vi "IMU garbo.vi"(5 "Align?":bool, 6 "Velocity Data":dbl[](array[numeric]), 7 "PID gains":T1={"proportional gain (Kc)"=1.0, "integral time (Ti, min)"=0.01, "derivative time (Td, min)"=0.0} {"derivative time (Td, min)" format="%.3f"; "integral time (Ti, min)" format="%.3f"; "proportional gain (Kc)" format="%.3f"}, 8 "Numeric":dbl, 9 "Angular Data (Relative)":dbl[](array[numeric]), 10 "Angle to Get":dbl, 11 "Iterations":dbl) -> (0 "Current Velocity":dbl, 1 "output":dbl, 2 "output 2":dbl, 3 "IPCed":dbl)   [LabVIEW 2019]
uses:
  <vilib>/addons/control/pid/pid.llb/PID (DBL).vi
  <vilib>/addons/control/pid/NI_PID_pid.lvlib
panel:
  out "Error":dbl
  out "Waveform Chart":cluster{"Current Angle 2":dbl, "Numeric":dbl}(graph)
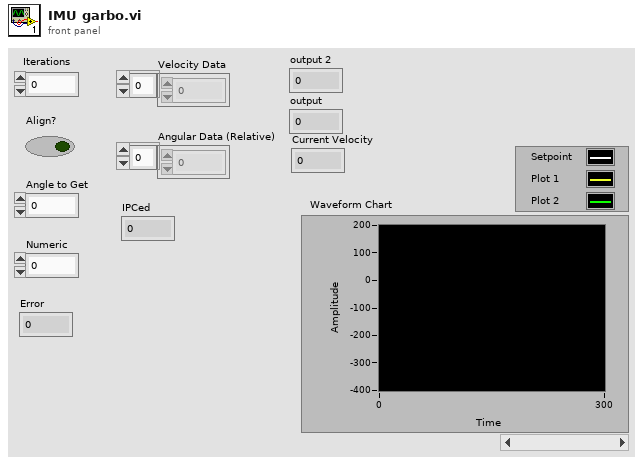
[diagram p1: front panel]
types:
  T1 = cluster{"proportional gain (Kc)":dbl, "integral time (Ti, min)":dbl, "derivative time (Td, min)":dbl}
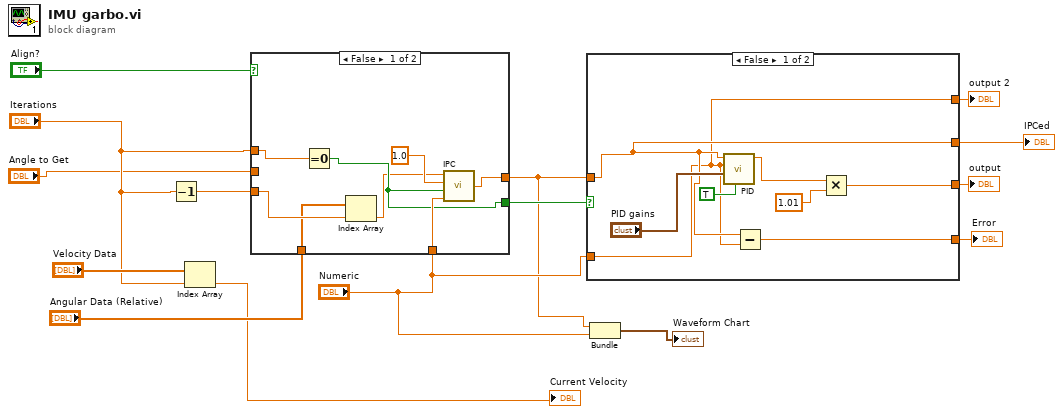
[diagram p0: block diagram]
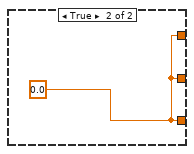
[diagram p2: hidden frame]
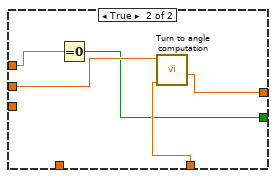
[diagram p3: hidden frame]
diagram:
  n1 = Decrement(x="Iterations") -> (x-1=w14:dbl)
  n2 = Index Array(array="Velocity Data", index="Iterations") -> (element=→"Current Velocity":dbl)
  n3 = case shown="False" "Align?" {
    tunnel: w14 -> [w22 _]
    tunnel: "Iterations" -> [w23 w28]
    tunnel: "Angle to Get" -> [_ w27]
    tunnel: "Angular Data (Relative)" -> [w21 _]
    tunnel: "Numeric" -> [w19 w26]
    tunnel: [w18 w25] -> w3
    tunnel: [w17 w24] -> w5
    frame False {
      n4 = Equal To 0?(x=w23) -> (x = 0?=w17:bool)
      n5 = Index Array(array=w21, index=w22) -> (element=w16:dbl)
      n6 = call "IPC.vi"("Initilization"=w19, "Reset"=w17, "Multiplier"=1.0, "Value"=w16) -> ("IPCed"=w18:dbl)  [unwired: 2 in]
    }
    frame True {
      n7 = Equal To 0?(x=w28) -> (x = 0?=w24:bool)
      n8 = call "Turn to angle computation.vi"("Current Angle"=w26, "Angle To Get"=w27) -> ("Current Angle 2"=w25:dbl)  [unwired: 9 in]
    }
  }
  n9 = case shown="False" w5 {
    tunnel: w3 -> [w31 _]
    tunnel: "Numeric" -> [w30 _]
    tunnel: [w31 w37] -> w9
    tunnel: [w30 w37] -> w8
    tunnel: [w33 w37] -> w7
    tunnel: [w29 _] -> w1
    frame False {
      n10 = call-poly <vilib>:"PID.vi"("reinitialize? (F)"=TRUE, "PID gains"="PID gains", "process variable"=w30, "setpoint"=w31) -> ("output"=w35:dbl)  [unwired: 6 in, 1 out]
      n11 = Subtract(x=w31, y=w30) -> (x-y=w29:dbl)
      n12 = Multiply(x=w35, y=1.01) -> (x*y=w33:dbl)
    }
    frame True {
      w37 = 0.0
    }
  }
  "IPCed" <- w9
  "output 2" <- w8
  "output" <- w7
  "Error" <- w1
  n13 = Bundle("Current Angle 2"=w3, "Numeric"="Numeric") -> (→"Waveform Chart":cluster{"Current Angle 2":dbl, "Numeric":dbl})  [unwired: 1 in]
